vi "List-Sort Item Names.vi"(9 "Separate Sign":string="-", 11 "List in":refnum<vi>) -> (3 "List Out":refnum<vi>)   [LabVIEW 2024]
uses:
  53475047-e612-412f-8000-13602b2c9e32.vi
  <vilib>/Comparison/Less/Less Functor/Less Functor.lvclass
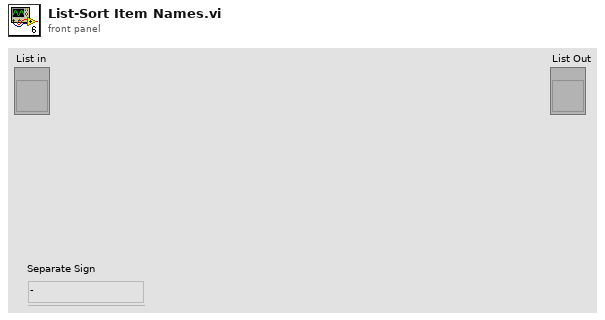
[diagram p1: front panel]
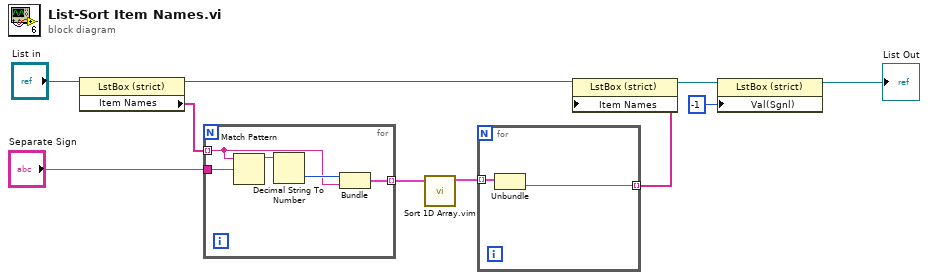
[diagram p0: block diagram]
diagram:
  n1 = property class="LstBox (strict)"(reference="List in") -> (reference out=w9:refnum<vi>, "Item Names"=w5:string[])  [unwired: 1 in, 1 out]
  n2 = for {
    tunnel: w5 -> [w12] mode=indexing
    tunnel: "Separate Sign" -> [w15]
    tunnel: [w11] -> w3 mode=indexing
    n3 = Match Pattern(string=w12, regular expression=w15) -> (before substring=w14:string)  [unwired: 1 in, 3 out]
    n4 = Decimal String To Number(string=w14) -> (number=w13:i32)  [unwired: 2 in, 1 out]
    n5 = Bundle(w13, w12) -> (w11:cluster{i32, string})  [unwired: 1 in]
  }
  n6 = call "Sort 1D Array.vim"("unsorted array"=w3) -> ("sorted array"=w2:cluster{i32, string}[])  [unwired: 10 in]
  n7 = for {
    tunnel: w2 -> [w17] mode=indexing
    tunnel: [w16] -> w1 mode=indexing
    n8 = Unbundle(w17) -> (w16:string)  [unwired: 1 out]
  }
  n9 = property class="LstBox (strict)"(reference=w9, "Item Names"=w1) -> (reference out=w8:refnum<vi>)  [unwired: 1 in, 1 out]
  n10 = property class="LstBox (strict)"(reference=w8, "Val(Sgnl)"=-1 ("Value")) -> (reference out=→"List Out":refnum<vi>)  [unwired: 1 in, 1 out]
